vi "User add Write.vi"(4 "error in (no error)":errorcluster, 5 "Value":bool, 6 "Container State":T6, 7 "Display State In":T1) -> (0 "error out":errorcluster, 3 "Display State Out":T1)   [LabVIEW 2020, in "KTable.xctl"]
uses:
  KTable.xctl
  <vilib>/_xctls/Container State.ctl
  State.ctl
  ColumnSpec.ctl
  ColumnType.ctl
  Table Properties.ctl
  Events.ctl
  Event Data.ctl
  Event Type.ctl
  <vilib>/_xctls/XControlSupport.lvlib
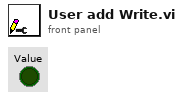
[diagram p1: front panel]
types:
  T1 = typedef "KTable.xctl/State.ctl" = cluster{"Columns":T2[], "Listbox":refnum<vi>, "Default row":string[], "Properties":T4, "Events":T5, "Locked":bool[][], "Size":cluster{"Rows":i32, "Columns":i32}, "rings":i32[][], "DefColors":u32[], "highlight row":bool}
  T2 = typedef "KTable.xctl/ColumnSpec.ctl" = cluster{"Name":string, "Type":T3, "Width":i32, "Strings":string[], "Position":enum16{"Left", "Center", "Right"}, "locked":bool, "cds":cluster{"Strings":string[]}[][], "Hide NaN":bool}
  T3 = typedef "KTable.xctl/ColumnType.ctl" = enum16{"String", "Enum", "Int", "Double", "Boolean", "Ring", "Formula", "Color"}
  T4 = typedef "KTable.xctl/Table Properties.ctl" = cluster{"Vertical scrollbar":bool, "User add/delete":bool, "Max rows":i32, "Row headers":bool}
  T5 = typedef "KTable.xctl/Events.ctl" = cluster{"Items Changed":refnum<user-event>}
  T6 = typedef "XControlSupport.lvlib/Container State.ctl" = cluster{"Indicator?":bool, "Run Mode?":bool, " Refnum":refnum<vi>}
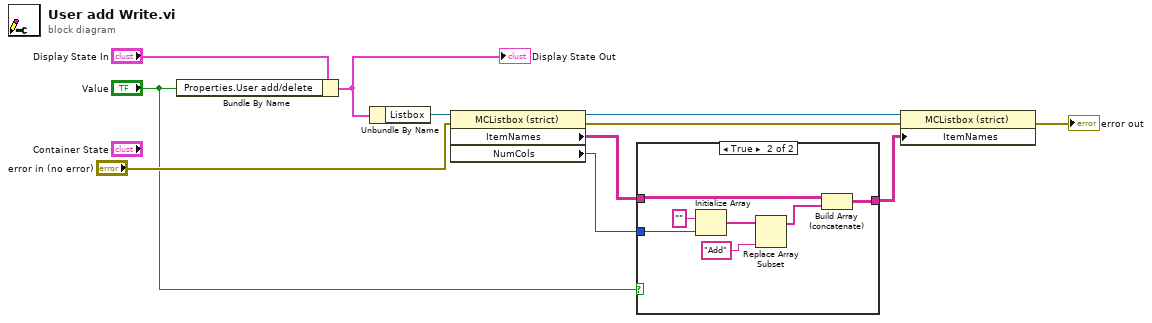
[diagram p0: block diagram]
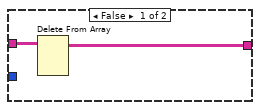
[diagram p2: hidden frame]
diagram:
  n1 = Bundle By Name(cluster="Display State In", "Properties.User add/delete"="Value") -> (w2:T1)
  "Display State Out" <- w2
  n2 = Unbundle By Name(w2) -> ("Listbox"=w10:refnum<vi>)
  n3 = property class="MCListbox (strict)"(reference=w10, error in="error in (no error)") -> (reference out=w9:refnum<vi>, error out=w7:errorcluster, "ItemNames"=w4:string[][], "NumCols"=w1:u32)
  n4 = case shown="True" "Value" {
    tunnel: w4 -> [w13 w16]
    tunnel: [w12 w14] -> w3
    tunnel: w1 -> [_ w17]
    frame False {
      n5 = Delete From Array(array=w13) -> (array with subset deleted=w12:string[][])  [unwired: 3 in, 1 out]
    }
    frame True {
      n6 = Initialize Array("" ("element"), w17) -> (w20:string[])
      n7 = Replace Array Subset(array=w20, new element="Add" ("new element/subarray")) -> (w15:string[])  [unwired: 1 in]
      n8 = Build Array (concatenate)(w16, w15) -> (w14:string[][])
    }
  }
  n9 = property class="MCListbox (strict)"(reference=w9, error in=w7, "ItemNames"=w3) -> (error out=→"error out":errorcluster)  [unwired: 1 out]
